vi "Read_Fast.vi"(8 "error in (no error)":errorcluster, 9 "Results Array In":dbl[](array[numeric]), 11 "SoftmotionAxis in":refnum<class "SoftmotionAxis.lvclass">) -> (0 "error out":errorcluster, 1 "appended array":dbl[](array[numeric]), 3 "SoftmotionAxis out":refnum<class "SoftmotionAxis.lvclass">)   [LabVIEW 2017, in "SoftmotionAxis.lvclass"]
uses:
  SoftmotionAxis.lvclass
  <resource>/objmgr/nimcai.rc
  <resource>/objmgr/nimotion.rc
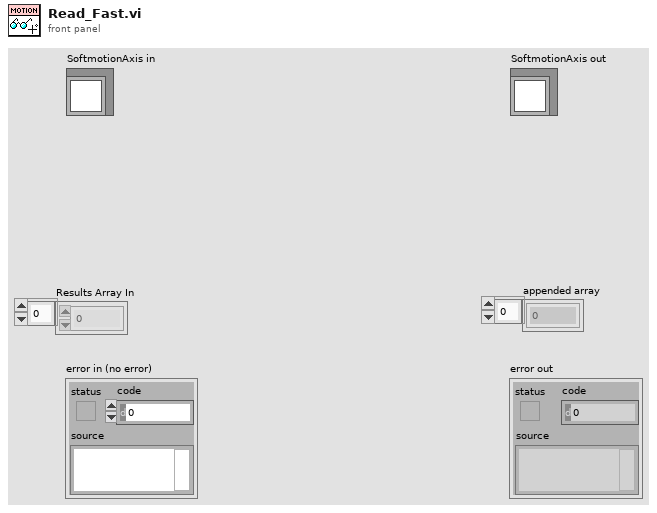
[diagram p1: front panel]
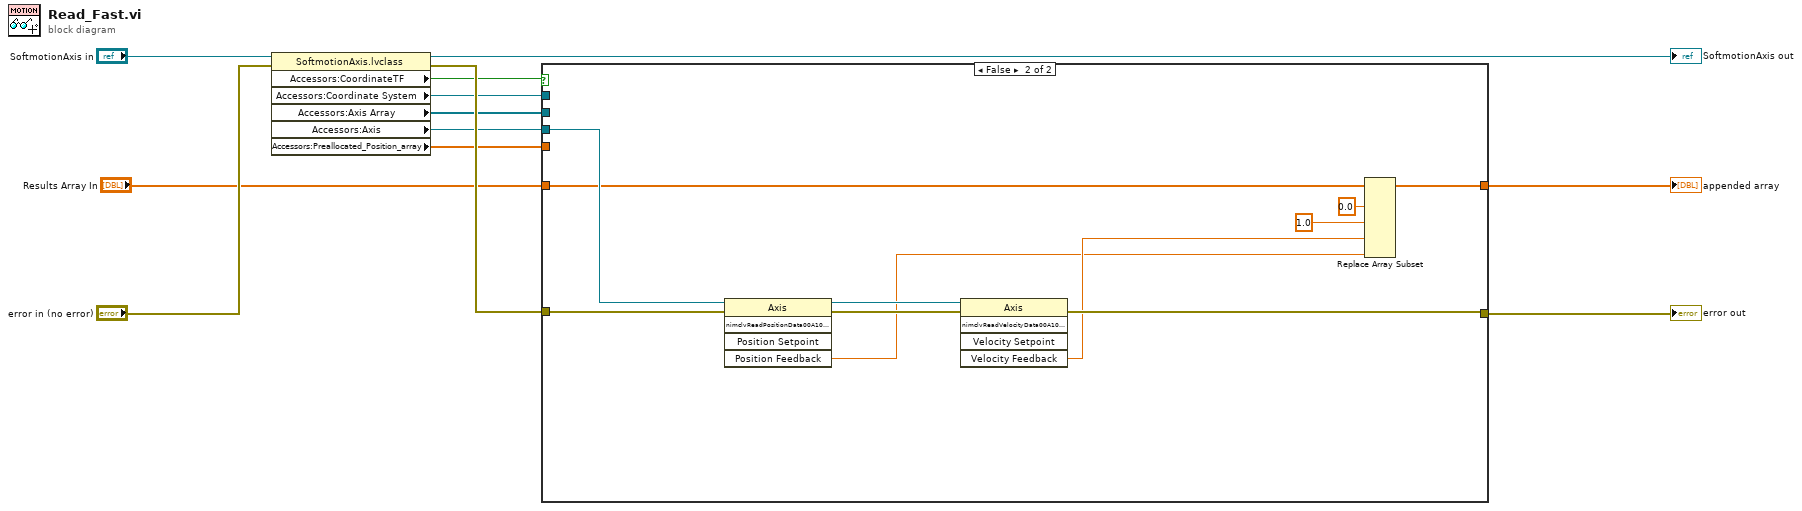
[diagram p0: block diagram]
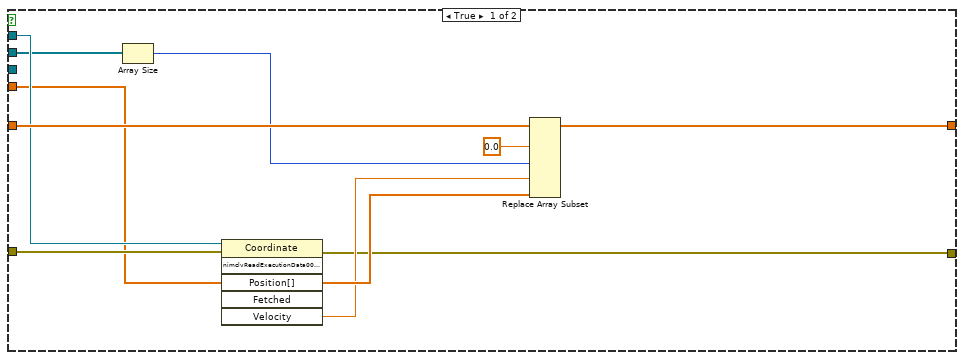
[diagram p2: hidden frame]
diagram:
  n1 = property class="SoftmotionAxis.lvclass"(reference="SoftmotionAxis in", error in="error in (no error)") -> (reference out=→"SoftmotionAxis out":refnum<class "SoftmotionAxis.lvclass">, error out=w7:errorcluster, "Accessors:CoordinateTF"=w4:bool, "Accessors:Coordinate System"=w3:refnum<k21>, "Accessors:Axis Array"=w5:refnum<k21>[], "Accessors:Axis"=w6:refnum<k21>, "Accessors:Preallocated_Position_array"=w2:dbl[])
  n2 = case shown="False" w4 {
    tunnel: [w22 w29] -> w9
    tunnel: [w17 w26] -> w12
    tunnel: w7 -> [w20 w34]
    tunnel: w6 -> [_ w31]
    tunnel: w3 -> [w21 _]
    tunnel: w5 -> [w14 _]
    tunnel: "Results Array In" -> [w23 w30]
    tunnel: w2 -> [w16 _]
    frame True {
      n3 = Array Size(array=w14) -> (size(s)=w13:i32)
      n4 = invoke class="Coordinate" method="nimclvReadExecutionData00A10011"(reference=w21, error in=w20, "Position[]"=w16) -> (error out=w17:errorcluster, "Position[]"=w19:dbl[], "Velocity"=w18:dbl)  [unwired: 3 in, 3 out]
      n5 = Replace Array Subset(array=w23, new element #1=0.0 ("new element/subarray"), new element #2=w13, new element #3=w18, new element #4=w19) -> (w22:dbl[])  [unwired: 4 in]
    }
    frame False {
      n6 = invoke class="Axis" method="nimclvReadPositionData00A10001"(reference=w31, error in=w34) -> (reference out=w33:refnum<k21>, error out=w32:errorcluster, "Position Feedback"=w24:dbl)  [unwired: 3 in, 2 out]
      n7 = invoke class="Axis" method="nimclvReadVelocityData00A10001"(reference=w33, error in=w32) -> (error out=w26:errorcluster, "Velocity Feedback"=w25:dbl)  [unwired: 3 in, 3 out]
      n8 = Replace Array Subset(array=w30, new element #1=0.0 ("new element/subarray"), new element #2=1.0 ("new element/subarray"), new element #3=w25, new element #4=w24) -> (w29:dbl[])  [unwired: 4 in]
    }
  }
  "error out" <- w12
  "appended array" <- w9
